vi "Close.vi"(8 "error in (no error)":errorcluster) -> (0 "Error Out":errorcluster, 3 "Return":i32)   [LabVIEW 2015]
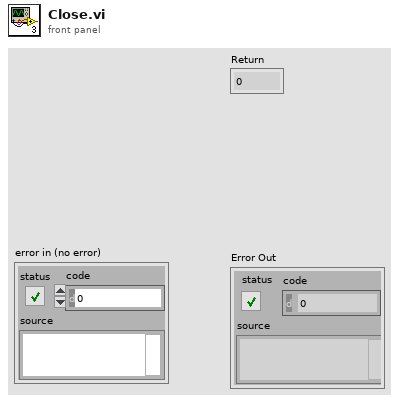
[diagram p1: front panel]
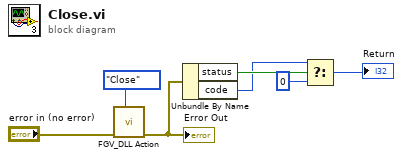
[diagram p0: block diagram]
diagram:
  n1 = call "FGV_DLL Action.vi"("State"=enum16{"Initial", "Run", "Close"}."Close", "Error In"="error in (no error)") -> ("Error Out"=w5:errorcluster)  [unwired: 9 in]
  "Error Out" <- w5
  n2 = Unbundle By Name(w5) -> ("status"=w4:bool, "code"=w3:i32)
  n3 = Select(t=w3, s=w4, f=0) -> (s? t:f=→"Return":i32)
